vi "Test Update Current Tool.vi"() -> ()   [LabVIEW 2011]
uses:
  WorkTable Class.lvclass
panel:
  in  "Tool 2":T1(ring)
  out "Tool Position 2":i32
  out "error out":errorcluster
  out "Tool Position":i32
  in  "Tool":T1(ring)
  in  "Config Folder":path=path "C:/Users/dustindam/Desktop/gantry/Config"
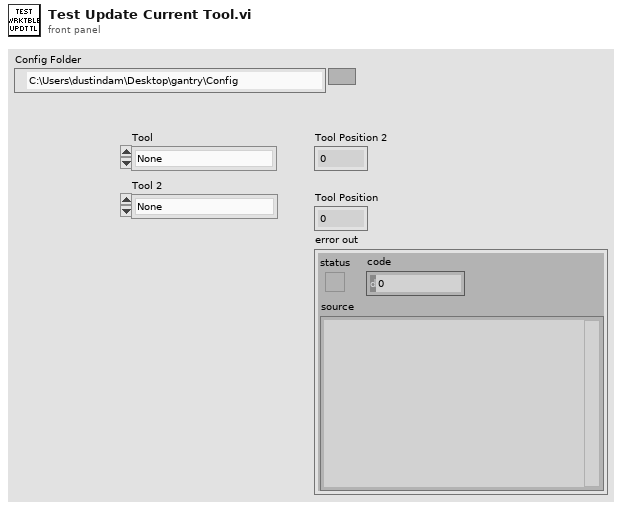
[diagram p1: front panel]
types:
  T1 = enum16{"None", "Grabber", "Picker", "Tool Setter"}
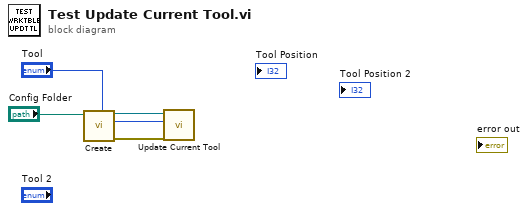
[diagram p0: block diagram]
diagram:
  n1 = call "Create.vi"("Config Folder"="Config Folder") -> ("error out"=w1:errorcluster, "WorkTable Class out"=w3:refnum<class "WorkTable Class.lvclass">)  [unwired: 9 in]
  n2 = call-dynamic "Update Current Tool.vi"("error in (no error)"=w1, "Tool"="Tool", "WorkTable Class in"=w3) -> ()  [unwired: 6 in, 3 out]
